vi "set_origin_by_name.vi"(8 "error in (no error)":errorcluster caption="错误输入（无错误）", 9 "new pos":dbl, 10 "name":string, 11 "MotorSystem 输入":refnum<class "MotorSystem.lvclass">) -> (0 "error out":errorcluster caption="错误输出", 3 "MotorSystem 输出":refnum<class "MotorSystem.lvclass">)   [LabVIEW 2016, in "MotionControl_UFO_3DOF.lvlib" / "MotorSystem.lvclass"]
uses:
  <userlib>/MotionControl_UFO_3DOF/MotorSystem/MotorSystem.lvclass
  <userlib>/MotionControl_UFO_3DOF/MotorSystem/MotorSystem.lvclass/MotorSystem.ctl
  <userlib>/MotionControl_UFO_3DOF/OneMotion/OneMotion.lvclass
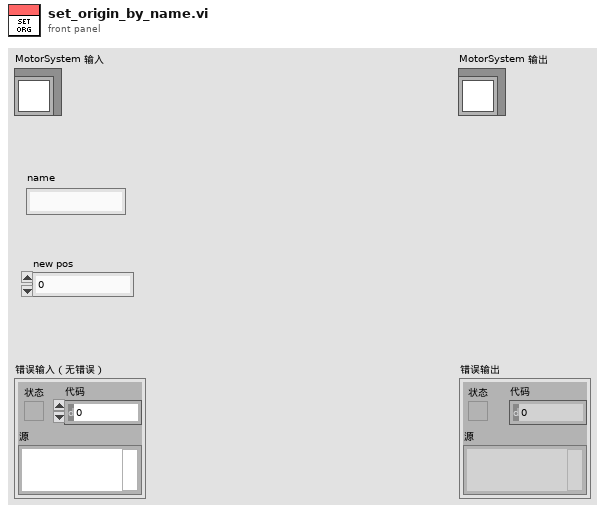
[diagram p1: front panel]
types:
  T1 = typedef "MotionControl_UFO_3DOF.lvlib/MotorSystem.lvclass/MotionCluster.ctl" = cluster{"OneMotion.lvclass":refnum<class "OneMotion.lvclass">, "connected?":bool, "default enabled?":bool, "enabled?":bool}
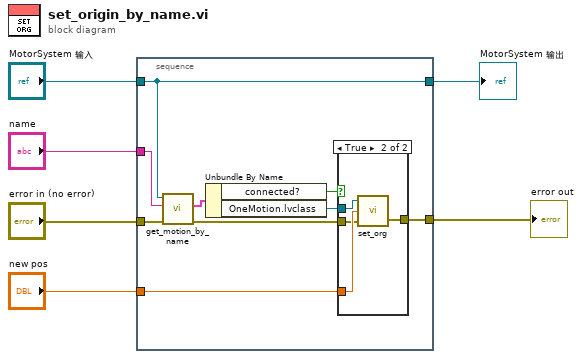
[diagram p0: block diagram]
diagram:
  n1 = stacked-sequence {
    tunnel: [w8] -> w6
    tunnel: [w15] -> w4
    tunnel: "MotorSystem 输入" -> [w15]
    tunnel: "error in (no error)" -> [w10]
    tunnel: "name" -> [w14]
    tunnel: "new pos" -> [w11]
    frame #0 {
      n2 = call <userlib>:"get_motion_by_name.vi"("error in (no error)"=w10, "name"=w14, "MotorSystem in"=w15) -> ("error out"=w9:errorcluster, "motion cluster"=w13:T1)  [unwired: 6 in, 1 out]
      n3 = Unbundle By Name(w13) -> ("connected?"=w7:bool, "OneMotion.lvclass"=w12:refnum<class "OneMotion.lvclass">)
      n4 = case shown="True" w7 {
        tunnel: w12 -> [_ w20]
        tunnel: w11 -> [_ w19]
        tunnel: w9 -> [w16 w18]
        tunnel: [w16 w17] -> w8
        frame False {
        }
        frame True {
          n5 = call <userlib>:"set_org.vi"("error in (no error)"=w18, "pos"=w19, "OneMotion 输入"=w20) -> ("error out"=w17:errorcluster)  [unwired: 1 out]
        }
      }
    }
  }
  "error out" <- w6
  "MotorSystem 输出" <- w4
